vi "POL.vi"(0 "System no.":i32=1 min=1 max=4 step=1, 2 "Axis":string[](array[string]), 3 "Polarization":T1(array[ring]), 5 "error in":errorcluster) -> (19 "error out":errorcluster)   [LabVIEW 2020]
doc: "Set axis to either 0% or 100% of its travel range. It does not use the previous history of the actuator but always uses the maximum number of pulses / maximum duration of pulses."
panel:
  # "Sets specified axis to either 0% or 100% of its travel range."
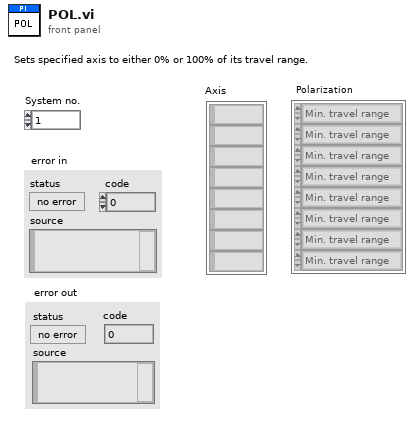
[diagram p1: front panel]
types:
  T1 = enum16{"Min. travel range", "Max. travel range"}[]
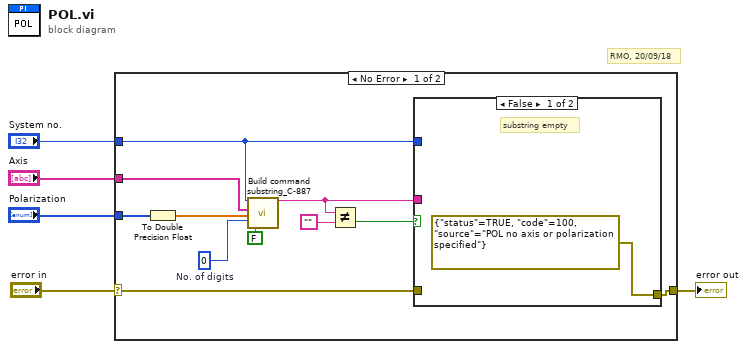
[diagram p0: block diagram]
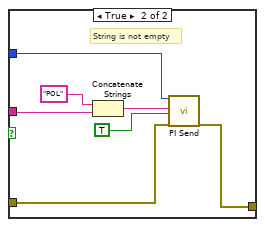
[diagram p2: hidden frame]
diagram:
  # "RMO, 20/09/18"
  n1 = case shown="No Error" "error in" {
    selector: "error in" -> [w9 w25]
    tunnel: [w16 w25] -> w5
    tunnel: "Polarization" -> [w8 _]
    tunnel: "System no." -> [w11 _]
    tunnel: "Axis" -> [w13 _]
    frame No Error {
      w6 = i16 0  # No. of digits
      n2 = To Double Precision Float(number=w8) -> (double precision float=w7:dbl[])
      n3 = call "Build command substring_C-887.vi"("System no."=w11, "Affected axes"=w13, "Parameters"=w7, "No. of digits"=w6, "Parameter no. format \n(Decimal: FALSE)"=FALSE ("Parameter no. format \n(Decimal: FALSE)")) -> ("Command substring"=w14:string)  [unwired: 2 in, 12 out]
      n4 = Not Equal?(x=w14, y="") -> (x != y?=w12:bool)
      n5 = case shown="False" w12 {
        tunnel: w14 -> [_ w23]
        tunnel: [errorcluster {"status"=TRUE, "code"=100, "source"="POL no axis or polarization specified"} ("error out") w19] -> w16
        tunnel: w9 -> [_ w20]
        tunnel: w11 -> [_ w18]
        frame False {
          # "substring empty"
        }
        frame True {
          # "String is not empty"
          n6 = Concatenate Strings("POL", w23) -> (w21:string)
          n7 = call "PI Send.vi"("System no."=w18, "String to send"=w21, "Attach termination char.?"=TRUE ("Attach Linefeed?"), "error in"=w20) -> ("error out"=w19:errorcluster)  [unwired: 2 in, 13 out]
        }
      }
    }
    frame Error {
    }
  }
  "error out" <- w5
